vi "ProgMon.Destroy.vi"(7 "Ignore Error":bool=TRUE, 8 "error in (no error)":errorcluster) -> (0 "error out":errorcluster)   [LabVIEW 2024, in "EQMF.lvlib" / "Status Utils.lvlib"]
uses:
  Status Utils.lvlib
  Queues/Q.Element.ctl
  Queues/Queue Utils.lvlib
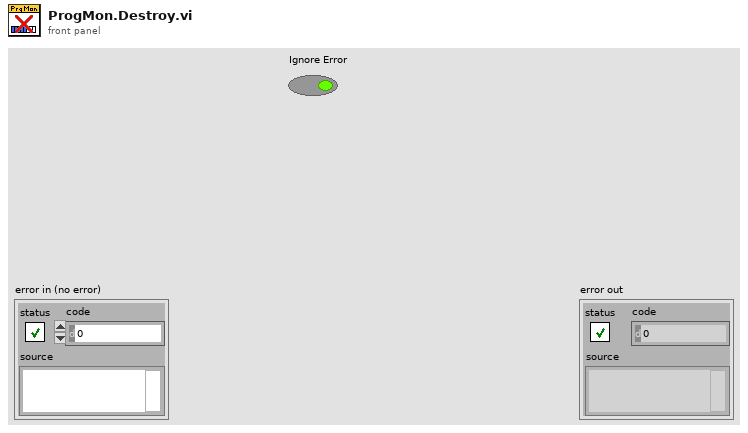
[diagram p1: front panel]
types:
  T1 = typedef "EQMF.lvlib/Queue Utils.lvlib/Q.Element.ctl" = cluster{"Cmd":string, "Sub":string, "Data1":variant, "Data2":variant}
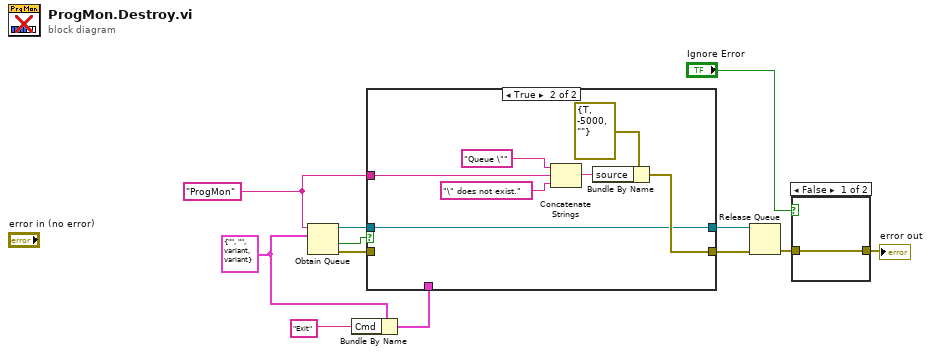
[diagram p0: block diagram]
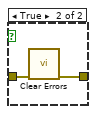
[diagram p2: hidden frame]
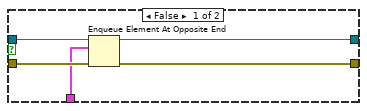
[diagram p3: hidden frame]
diagram:
  w4 = T1 {"Cmd"="", "Sub"="", "Data1"=variant, "Data2"=variant} ("Queue Element")
  w5 = "ProgMon" ("name (unnamed)")
  n1 = Obtain Queue(name (unnamed)=w5, element data type=w4) -> (queue out=w11:refnum<queue>, created new?=w10:bool, error out=w12:errorcluster)  [unwired: 3 in]
  n2 = Bundle By Name(cluster=w4, "Cmd"="Exit") -> (w8:T1)
  n3 = case shown="True" w10 {
    tunnel: w12 -> [w16 _]
    tunnel: w11 -> [w17 w18]
    tunnel: [w13 w20] -> w7
    tunnel: w5 -> [_ w19]
    tunnel: w8 -> [w15 _]
    tunnel: [w14 w18] -> w6
    frame False {
      n4 = Enqueue Element At Opposite End(queue=w17, element=w15, error in (no error)=w16) -> (queue out=w14:refnum<queue>, error out=w13:errorcluster)  [unwired: 1 in, 1 out]
    }
    frame True {
      n5 = Concatenate Strings("Queue \"", w19, "\" does not exist.") -> (w21:string)
      n6 = Bundle By Name(cluster=errorcluster {"status"=TRUE, "code"=-5000, "source"=""} ("error constant"), "source"=w21) -> (w20:errorcluster)
    }
  }
  n7 = Release Queue(queue=w6, error in (no error)=w7) -> (error out=w3:errorcluster)  [unwired: 1 in, 2 out]
  n8 = case shown="False" "Ignore Error" {
    tunnel: w3 -> [w25 w27]
    tunnel: [w25 w26] -> w2
    frame False {
    }
    frame True {
      n9 = call <vilib>:"Clear Errors.vi"("error in (no error)"=w27) -> ("error out"=w26:errorcluster)  [unwired: 5 in, 1 out]
    }
  }
  "error out" <- w2
